vi "Auto-Place lvl 1.vi"   [LabVIEW 2018]
uses:
  Implementation/Drive Operations.ctl
  <vilib>/Rock Robotics/Network Tables/NT Read Number.vi
  Framework/Robot Global Data.vi
types:
  T1 = cluster{"Reverse (T) / Normal (F)":bool, "Power Scaling (1=Normal) ":dbl, "Deadband Value":dbl}
  T2 = typedef "Drive Operations.ctl" = enum16{"Reserve", "Read Current", "Immediate", "J-Turn", "Play Back From Log", "Auto-Align"}
  T3 = typedef "Command Status Info.ctl" = cluster{"Name":string, "Status":T4, "notifier out":T5}
  T4 = typedef "Completion Status.ctl" = enum16{"Successful", "Aborted", "Incomplete"}
  T5 = typedef "Completion Notifier.ctl" = refnum<notifier>
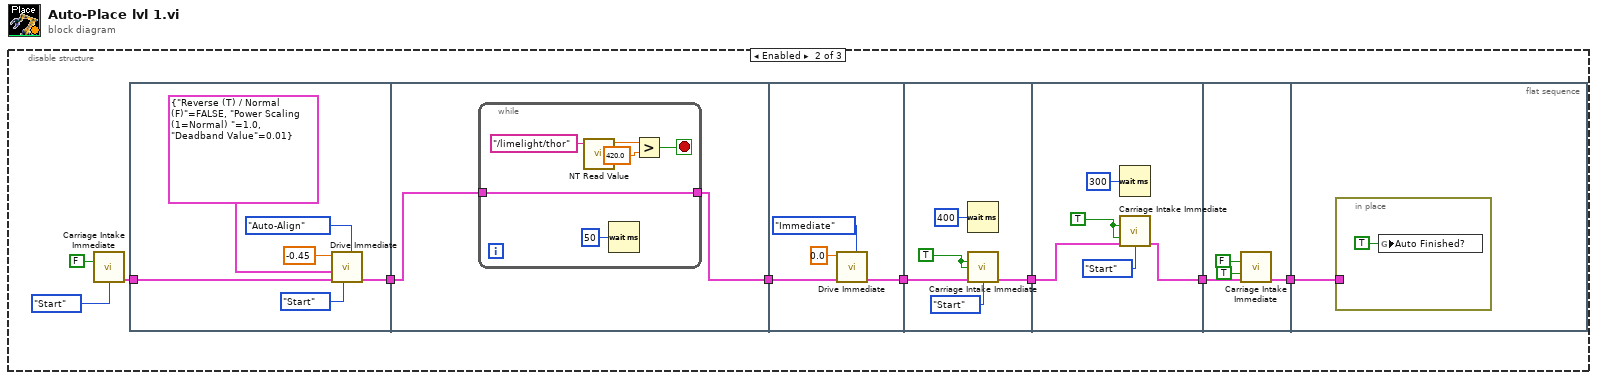
[diagram p0: block diagram]
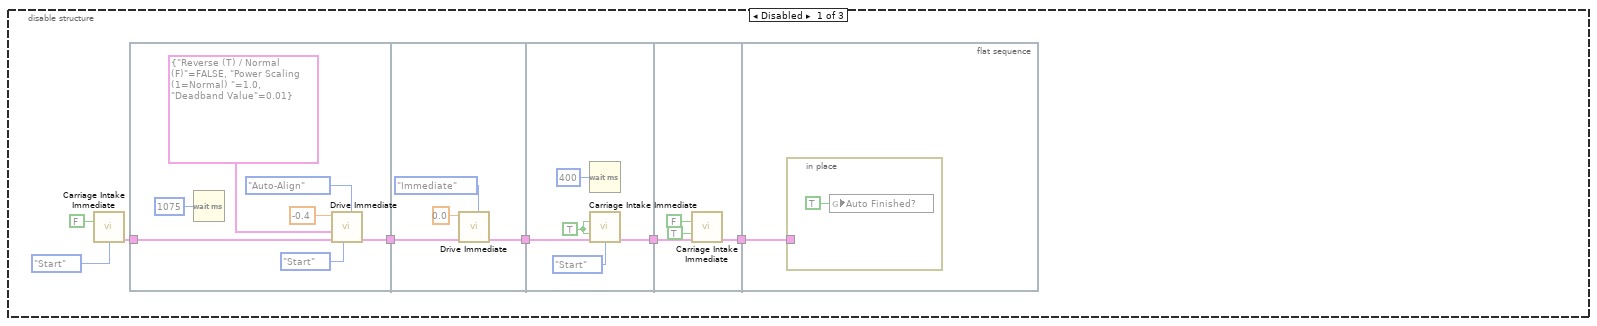
[diagram p2: hidden frame]
diagram:
  n1 = disable-structure shown="Enabled" {
    frame Disabled {
      n2 = call "Carriage Intake Immediate.vi"("Extend"=FALSE, "Synchronication"=enum16{"Start", "Wait"}."Start") -> ("Command Info Out"=w3:T3)  [unwired: 13 in]
      n3 = flat-sequence {
        tunnel: w3 -> [w11]
        tunnel: [w9] -> w7
        tunnel: w7 -> [w18]
        tunnel: [w17] -> w6
        tunnel: w6 -> [w23]
        tunnel: [w22] -> w5
        tunnel: w5 -> [w27]
        tunnel: [w25] -> w4
        tunnel: w4 -> [w28]
        frame #0 {
          n4 = Wait (ms)(milliseconds to wait=u32 1075) -> ()  [unwired: 1 out]
          n5 = call "Drive Immediate.vi"("Operation"=Drive_Operations."Auto-Align", "Synchronication"=enum16{"Start", "Wait"}."Start", "Command Info In"=w11, "Modifiers"=T1 {"Reverse (T) / Normal (F)"=FALSE, "Power Scaling (1=Normal) "=1.0, "Deadband Value"=0.01}, "Left Setpoint (Power)"=-0.4) -> ("Command Info Out"=w9:T3)  [unwired: 6 in]
        }
        frame #1 {
          n6 = call "Drive Immediate.vi"("Operation"=Drive_Operations."Immediate", "Command Info In"=w18, "Left Setpoint (Power)"=0.0) -> ("Command Info Out"=w17:T3)  [unwired: 8 in]
        }
        frame #2 {
          w19 = TRUE ("Extend")
          n7 = Wait (ms)(milliseconds to wait=u32 400) -> ()  [unwired: 1 out]
          n8 = call "Carriage Intake Immediate.vi"("Extend"=w19, "Close"=w19, "Command Info In"=w23, "Synchronication"=enum16{"Start", "Wait"}."Start") -> ("Command Info Out"=w22:T3)  [unwired: 11 in]
        }
        frame #3 {
          n9 = call "Carriage Intake Immediate.vi"("Extend"=FALSE, "Close"=TRUE, "Command Info In"=w27) -> ("Command Info Out"=w25:T3)  [unwired: 12 in]
        }
        frame #4 {
          n10 = in-place {
            in-place-border: w28 -> [_]
            n11 = global write "Robot Global Data.vi" "Auto Finished?"(TRUE ("Auto Finished?")) -> ()
          }
        }
      }
    }
    frame Enabled {
      n12 = call "Carriage Intake Immediate.vi"("Extend"=FALSE, "Synchronication"=enum16{"Start", "Wait"}."Start") -> ("Command Info Out"=w36:T3)  [unwired: 13 in]
      n13 = flat-sequence {
        tunnel: w36 -> [w41]
        tunnel: [w39] -> w33
        tunnel: w33 -> [w46]
        tunnel: [w45] -> w32
        tunnel: w32 -> [w56]
        tunnel: [w55] -> w38
        tunnel: w38 -> [w61]
        tunnel: [w60] -> w31
        tunnel: w31 -> [w64]
        tunnel: [w63] -> w30
        tunnel: w30 -> [w70]
        tunnel: [w68] -> w37
        tunnel: w37 -> [w71]
        frame #0 {
          n14 = call "Drive Immediate.vi"("Operation"=Drive_Operations."Auto-Align", "Synchronication"=enum16{"Start", "Wait"}."Start", "Command Info In"=w41, "Modifiers"=T1 {"Reverse (T) / Normal (F)"=FALSE, "Power Scaling (1=Normal) "=1.0, "Deadband Value"=0.01}, "Left Setpoint (Power)"=-0.45) -> ("Command Info Out"=w39:T3)  [unwired: 6 in]
        }
        frame #1 {
          n15 = while {
            tunnel: [w52] -> w45
            tunnel: w46 -> [w52]
            stop <- w48 stop-if-true
            n16 = call-poly <vilib>:"NT Read Value.vi"("Name"="/limelight/thor") -> ("Numeric"=w50:dbl)  [unwired: 9 in, 1 out]
            n17 = Wait (ms)(milliseconds to wait=u32 50) -> ()  [unwired: 1 out]
            n18 = Greater?(x=w50, y=420.0) -> (0:w48:bool)
          }
        }
        frame #2 {
          n19 = call "Drive Immediate.vi"("Operation"=Drive_Operations."Immediate", "Command Info In"=w56, "Left Setpoint (Power)"=0.0) -> ("Command Info Out"=w55:T3)  [unwired: 8 in]
        }
        frame #3 {
          w57 = TRUE ("Extend")
          n20 = Wait (ms)(milliseconds to wait=u32 400) -> ()  [unwired: 1 out]
          n21 = call "Carriage Intake Immediate.vi"("Extend"=w57, "Open"=w57, "Command Info In"=w61, "Synchronication"=enum16{"Start", "Wait"}."Start") -> ("Command Info Out"=w60:T3)  [unwired: 11 in]
        }
        frame #4 {
          w62 = TRUE ("Extend")
          n22 = Wait (ms)(milliseconds to wait=u32 300) -> ()  [unwired: 1 out]
          n23 = call "Carriage Intake Immediate.vi"("Extend"=w62, "Close"=w62, "Command Info In"=w64, "Synchronication"=enum16{"Start", "Wait"}."Start") -> ("Command Info Out"=w63:T3)  [unwired: 11 in]
        }
        frame #5 {
          n24 = call "Carriage Intake Immediate.vi"("Extend"=FALSE, "Close"=TRUE, "Command Info In"=w70) -> ("Command Info Out"=w68:T3)  [unwired: 12 in]
        }
        frame #6 {
          n25 = in-place {
            in-place-border: w71 -> [_]
            n26 = global write "Robot Global Data.vi" "Auto Finished?"(TRUE ("Auto Finished?")) -> ()
          }
        }
      }
    }
    frame Disabled {
    }
  }
